vi "FTW-Container-Construct.vi"(5 "LabVIEW Data Structure":variant, 11 "error in":errorcluster) -> (4 "Container":refnum<class "FTW-Container.lvclass">, 15 "error out":errorcluster)   [LabVIEW 2014, in "FTW-Container.lvclass"]
uses:
  FTW-Container.lvclass
panel:
  # "Inputs"
  # "Outputs"
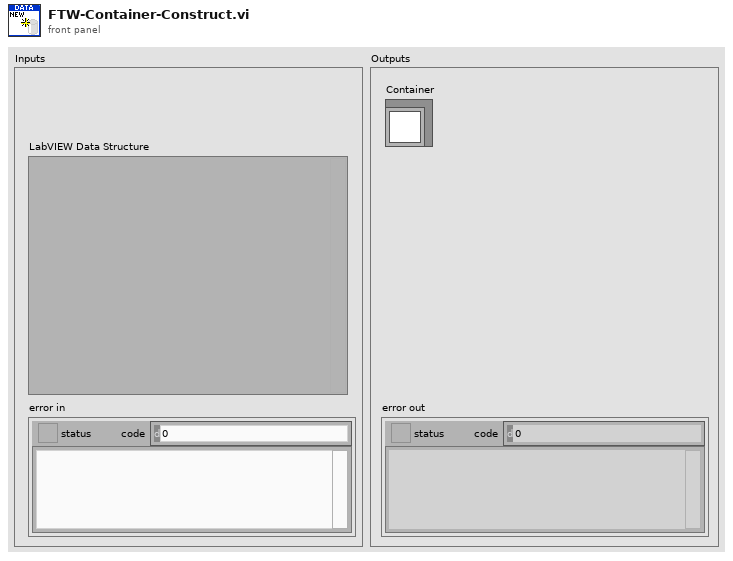
[diagram p1: front panel]
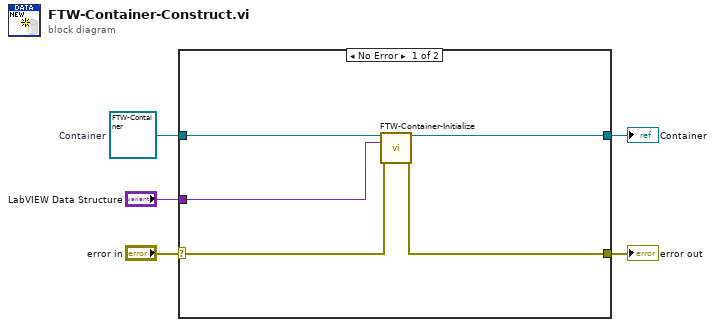
[diagram p0: block diagram]
diagram:
  w2 = refnum<class "FTW-Container.lvclass"> refnum  # Container
  n1 = case shown="No Error" "error in" {
    selector: "error in" -> [w8 w12]
    tunnel: [w7 w12] -> w5
    tunnel: [w9 w11] -> w3
    tunnel: w2 -> [w10 w11]
    tunnel: "LabVIEW Data Structure" -> [w6 _]
    frame No Error {
      n2 = call-dynamic "FTW-Container-Initialize.vi"("Container"=w10, "LabVIEW Data Structure"=w6, "error in"=w8) -> ("Container out"=w9:refnum<class "FTW-Container.lvclass">, "error out"=w7:errorcluster)  [unwired: 11 in]
    }
    frame Error {
    }
  }
  "error out" <- w5
  "Container" <- w3
